vi "GNSS RF Test Get InstDriver Handle.vi"(8 "error in (no error)":errorcluster, 11 "niDTS GNSS RF Test in":refnum<class "niDTS GNSS RF Test.lvclass">) -> (0 "error out":errorcluster, 2 "RiviInstDriver Handle in":T1, 3 "niDTS GNSS RF Test out":refnum<class "niDTS GNSS RF Test.lvclass">)   [LabVIEW 2015, in "niDTS GNSS.lvlib" / "niDTS GNSS RF Test.lvclass"]
uses:
  niDTS GNSS RF Test.lvclass
  RiviInstDriver/InstDriver/Includes/niInstDriver INC Handle.ctl
  RiviInstDriver/InstDriver/Objects/InstDriver.lvclass
  niDTS GNSS RF Test.lvclass/niDTS GNSS RF Test.ctl
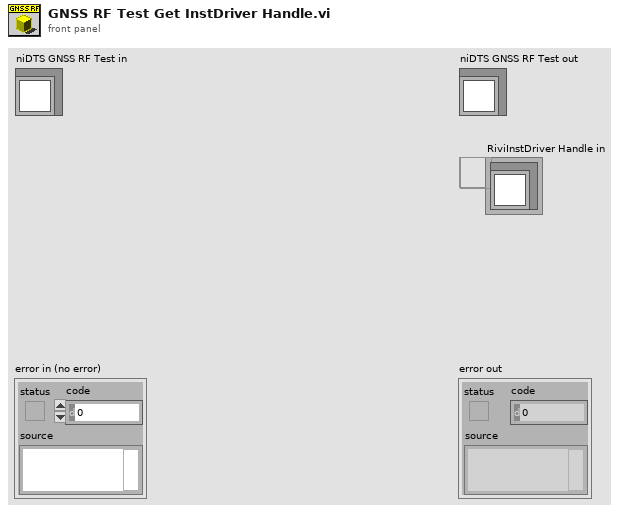
[diagram p1: front panel]
types:
  T1 = typedef "InstDriver.lvclass/niInstDriver INC Handle.ctl" = refnum<data-value>
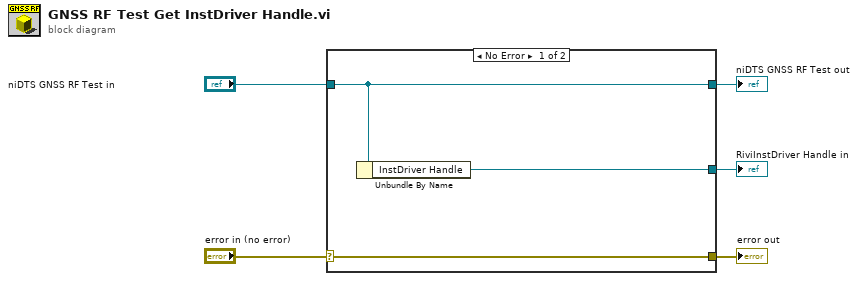
[diagram p0: block diagram]
diagram:
  n1 = case shown="No Error" "error in (no error)" {
    selector: "error in (no error)" -> [w8 w9]
    tunnel: [w8 w9] -> w4
    tunnel: [w7 w10] -> w2
    tunnel: "niDTS GNSS RF Test in" -> [w7 w10]
    tunnel: [w6 _] -> w1
    frame No Error {
      n2 = Unbundle By Name(w7) -> ("InstDriver Handle"=w6:T1)
    }
    frame Error {
    }
  }
  "error out" <- w4
  "niDTS GNSS RF Test out" <- w2
  "RiviInstDriver Handle in" <- w1
